vi "Read External Temp.vi"(8 "error in (no error)":errorcluster, 11 "VISA session":refnum<visa-resource-name>) -> (0 "error out":errorcluster, 2 "External PT100 Temperature":dbl format="%.2f", 3 "dup VISA session":refnum<visa-resource-name>)   [LabVIEW 2018, in "Lauda TCU.lvlib"]
uses:
  Lauda TCU.lvlib
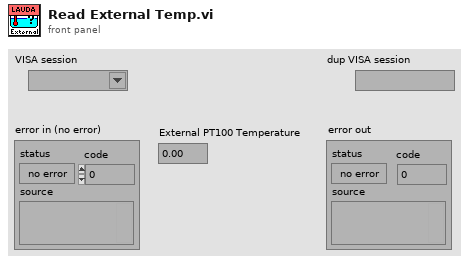
[diagram p1: front panel]
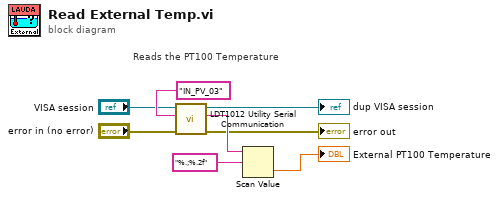
[diagram p0: block diagram]
diagram:
  # "Reads the PT100 Temperature"
  n1 = call "LDT1012 Utility Serial Communication.vi"("error in (no error)"="error in (no error)", "Command String"="IN_PV_03", "VISA session"="VISA session") -> ("error out"=→"error out":errorcluster, "Returned String"=w8:string, "dup VISA session"=→"dup VISA session":refnum<visa-resource-name>)  [unwired: 5 in, 1 out]
  n2 = Scan Value(string=w8, format string="%.;%.2f") -> (value=→"External PT100 Temperature":dbl)  [unwired: 1 in, 1 out]
